vi "Get Type.vi"(11 "Test Executive 1D in":refnum<class "Test Executive 1D.lvclass">) -> (3 "Type":string)   [LabVIEW 2017, in "Custom Type Test Executive.lvlib" / "Test Executive 1D.lvclass"]
uses:
  <vilib>/gpm_packages/@cs/test-executive/Source/Custom Type Test Executive/Test Executive 1D Data Type/Test Executive 1D.lvclass
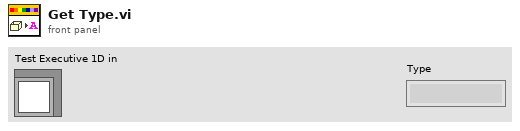
[diagram p1: front panel]
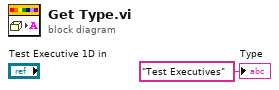
[diagram p0: block diagram]
diagram:
  "Type" <- "Test Executives" ("Type")
